vi "CAN_LIN_FlexRay_Configuration_Save.vi"(7 "path":path, 8 "error in (no error)":errorcluster caption="错误输入（无错误）", 9 "Config Name":string, 10 "Read/Write":enum16{"Read", "Write"}(ring), 11 "Data":T1={"Communication message"={"Sender"="", "receiver"="", "message"="", "data"=variant}, "Receive data"="", "error in"={"status"=FALSE, "code"=0, "source"=""}, "Data"={"DLL_PATH"=path "", "Call Array"=["CAN_Demo0", "LIN_Demo0"], "Project_PATH"=path ""}, "AsynCall?"=FALSE}) -> (0 "error in (no error)":errorcluster caption="错误输入（无错误）", 2 "path out":path, 3 "Data out":T1={"Communication message"={"Sender"="", "receiver"="", "message"="", "data"=variant}, "Receive data"="", "error in"={"status"=FALSE, "code"=0, "source"=""}, "Data"={"DLL_PATH"=path "", "Call Array"=["CAN_Demo0", "LIN_Demo0"], "Project_PATH"=path ""}, "AsynCall?"=FALSE})   [LabVIEW 2014]
uses:
  TypDef/CAN_LIN_FlexRay_Data.ctl
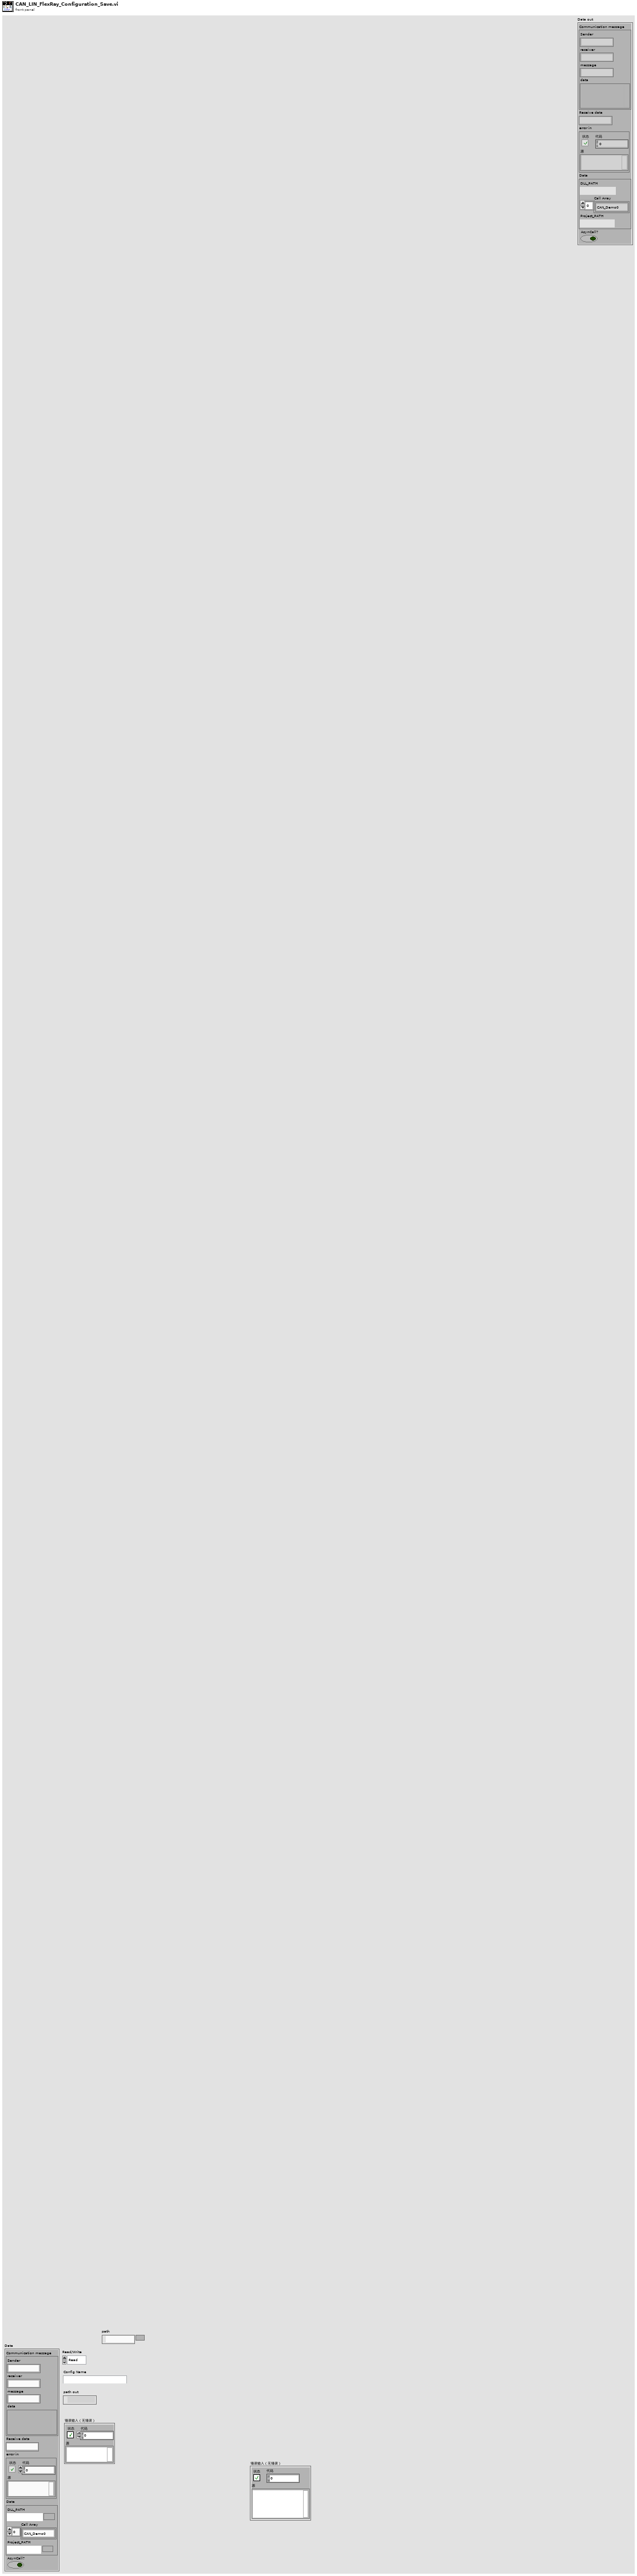
[diagram p1: front panel]
types:
  T1 = typedef "CAN_LIN_FlexRay_Data.ctl" = cluster{"Communication message":cluster{"Sender":string, "receiver":string, "message":string, "data":variant}, "Receive data":string, "error in":errorcluster, "Data":cluster{"DLL_PATH":path, "Call Array":string[], "Project_PATH":path}, "AsynCall?":bool}
  T2 = enum16{"open", "replace", "create", "open or create", "replace or create", "replace or create with confirmation"}
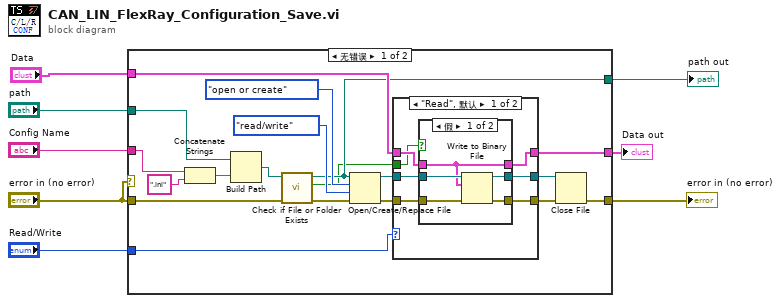
[diagram p0: block diagram]
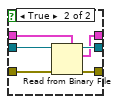
[diagram p2: hidden frame]
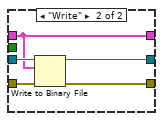
[diagram p3: hidden frame]
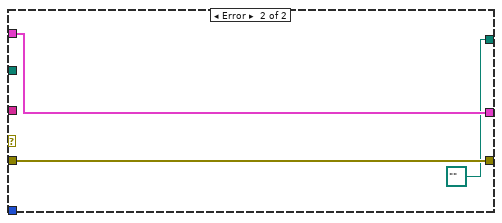
[diagram p4: hidden frame]
diagram:
  n1 = case shown="无错误" "error in (no error)" {
    tunnel: "Data" -> [w27 w52]
    tunnel: "Read/Write" -> [w20 _]
    tunnel: [w19 w52] -> w1
    tunnel: [w18 w53] -> w7
    tunnel: "error in (no error)" -> [w12 w53]
    tunnel: [w13 path "" ("appended path")] -> w6
    tunnel: "Config Name" -> [w16 _]
    tunnel: "path" -> [w9 _]
    frame No Error {
      n2 = Concatenate Strings(w16, ".ini") -> (w15:string)
      n3 = Build Path(base path=w9, name or relative path=w15) -> (appended path=w14:path)
      n4 = call <vilib>:"Check if File or Folder Exists.vi"("error in (no error)"=w12, "path"=w14) -> ("error out"=w11:errorcluster, "file or folder exists?"=w10:bool, "dup path"=w13:path)  [unwired: 7 in]
      n5 = Open/Create/Replace File(file path (use dialog)=w13, error in=w11, operation (0:open)=T2."open or create" ("操作(0:open)"), access (0:read/write)=enum16{"read/write", "read-only", "write-only"}."read/write" ("权限(0:read/write)")) -> (refnum out=w24:refnum<file>, error out=w23:errorcluster)  [unwired: 2 in, 1 out]
      n6 = case shown="\"Read\", 默认" w20 {
        tunnel: w27 -> [w31 w46]
        tunnel: w24 -> [w34 w50]
        tunnel: w23 -> [w29 w49]
        tunnel: [w33 w48] -> w22
        tunnel: [w32 w47] -> w21
        tunnel: [w30 w46] -> w19
        tunnel: w10 -> [w28 _]
        frame "Read", Default {
          n7 = case shown="假" w28 {
            tunnel: w34 -> [w37 w45]
            tunnel: w29 -> [w39 w44]
            tunnel: [w36 w43] -> w33
            tunnel: [w38 w42] -> w32
            tunnel: w31 -> [w35 w41]
            tunnel: [w35 w40] -> w30
            frame False {
              n8 = Write to Binary File(file (use dialog)=w37, data=w35, error in=w39) -> (refnum out=w36:refnum<file>, error out=w38:errorcluster)  [unwired: 3 in, 1 out]
            }
            frame True {
              n9 = Read from Binary File(5:w41, 8:w44, 11:w45) -> (0:w42:errorcluster, 2:w40:T1, 3:w43:refnum<file>)  [unwired: 3 in, 1 out]
            }
          }
        }
        frame "Write" {
          n10 = Write to Binary File(file (use dialog)=w50, data=w46, error in=w49) -> (refnum out=w48:refnum<file>, error out=w47:errorcluster)  [unwired: 3 in, 1 out]
        }
      }
      n11 = Close File(refnum=w22, error in=w21) -> (error out=w18:errorcluster)  [unwired: 1 out]
    }
    frame Error {
    }
  }
  "error in (no error)" <- w7
  "path out" <- w6
  "Data out" <- w1
